vi "init pcan.vi"(8 "error in (no error)":errorcluster) -> (0 "error out":errorcluster, 3 "function return":i32)   [LabVIEW 2024, in "libsocketcan_fd.lvlib"]
doc: "int init_pcan(void);"
uses:
  <userlib>/libsocketcan_fd/libsocketcan_fd.lvlib
  home/lvuser/natinst/bin/libsocketcan_fd.so
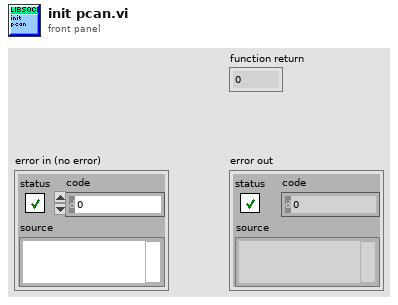
[diagram p1: front panel]
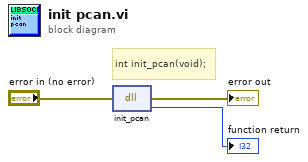
[diagram p0: block diagram]
diagram:
  # "int init_pcan(void);"
  n1 = dll-call lib="home/lvuser/natinst/bin/libsocketcan_fd.so" fn="init_pcan"(error in="error in (no error)") -> (error out=→"error out":errorcluster, "return type"=→"function return":i32)  [unwired: 2 in, 1 out]
